vi "Update Waypoint Marker Position.vi"(8 "Error In":errorcluster, 10 "index":i32, 11 "This VI":refnum<vi>) -> (0 "error out":errorcluster)   [LabVIEW 2014]
uses:
  C:/Robotic Systems/Products/AgFalcon/Software/Ground Station/Data/Mapping DLL/GMap.NET.WindowsForms.dll
  Data/Mapping DLL/GMap.NET.WindowsForms.dll
  Reference/SubVI/Main Map Control Refernce.vi
  Missions/FGVs/Virtual Waypoints/Methods/Get Selected Virtual WP.vi
  Missions/FGVs/Virtual Waypoints/Methods/Set Selected Virtual WP.vi
  Reference/SubVI/GMap DLL Refernce.vi
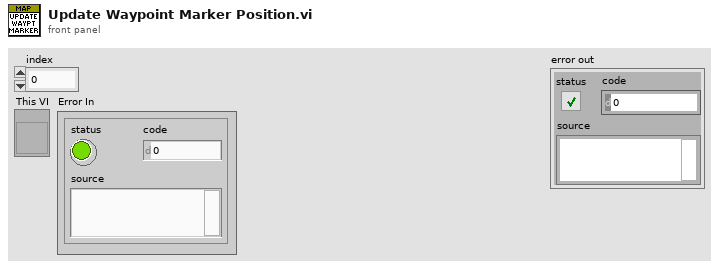
[diagram p1: front panel]
types:
  T1 = typedef "Virtual Waypoint.ctl" = cluster{"Waypoint Type":T2, "Lat":sgl, "Lon":sgl, "Altitude (m)":sgl, "Inspection Height (m)":sgl, "Circumnavigate Radius (m)":sgl, "Grid Waypoint?":bool, "Capture Photo":bool, "Speed (m/s)":sgl}
  T2 = typedef "Waypoint Type.ctl" = enum16{"PASS-THROUGH", "INSPECT", "CIRCUMNAVIGATE"}
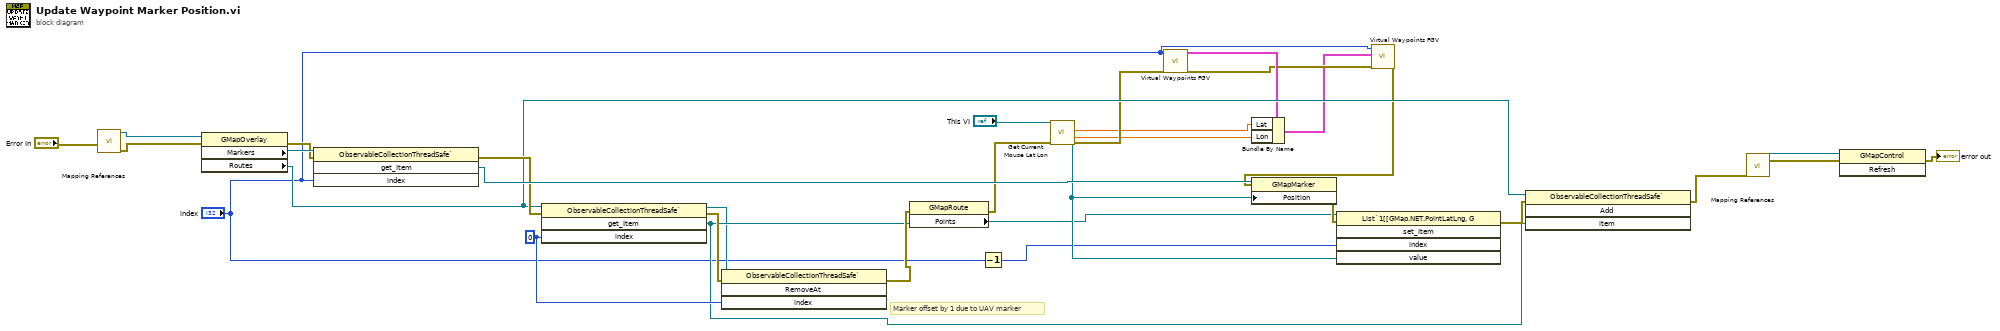
[diagram p0: block diagram]
diagram:
  w18 = 0 ("index")
  # "Marker offset by 1 due to UAV marker"
  n1 = call-poly "Mapping References.vi"("Error In"="Error In") -> ("Error Out"=w31:errorcluster, "Main Map Reference"=w32:refnum<k24>)  [unwired: 9 in]
  n2 = property class="GMapOverlay"(reference=w32, error in=w31) -> (error out=w29:errorcluster, "Markers"=w30:refnum<k24>, "Routes"=w9:refnum<k24>)  [unwired: 1 out]
  n3 = invoke class="ObservableCollectionThreadSafe`" method="get_Item"(reference=w30, error in=w29, "index"="index") -> (error out=w25:errorcluster, "get_Item"=w26:refnum<k24>)  [unwired: 1 in, 2 out]
  n4 = invoke class="ObservableCollectionThreadSafe`" method="get_Item"(reference=w9, error in=w25, "index"=w18) -> (reference out=w10:refnum<k24>, error out=w14:errorcluster, "get_Item"=w11:refnum<k24>)  [unwired: 1 in, 1 out]
  n5 = invoke class="ObservableCollectionThreadSafe`" method="RemoveAt"(reference=w10, error in=w14, "index"=w18) -> (error out=w17:errorcluster)  [unwired: 1 in, 3 out]
  n6 = property class="GMapRoute"(reference=w11, error in=w17) -> (error out=w24:errorcluster, "Points"=w21:refnum<k24>)  [unwired: 1 out]
  n7 = Decrement(x="index") -> (x-1=w20:i32)
  n8 = call "Get Current Mouse Lat Lon.vi"("error in (no error)"=w24, "This VI"="This VI") -> ("Error Out"=w8:errorcluster, "Lon"=w5:dbl, "Lat"=w6:dbl, "Point Ref"=w22:refnum<k24>)  [unwired: 6 in]
  n9 = call-poly "Virtual Waypoints FGV.vi"("Error In"=w8, "Waypoint Number"="index") -> ("Error Out"=w3:errorcluster, "Virtual Waypoint out"=w7:T1)  [unwired: 8 in]
  n10 = Bundle By Name(cluster=w7, "Lat"=w6, "Lon"=w5) -> (w2:T1)
  n11 = call-poly "Virtual Waypoints FGV.vi"("Error In"=w3, "Virtual Waypoints In"=w2, "Waypoint Index"="index") -> ("Error Out"=w1:errorcluster)  [unwired: 8 in]
  n12 = property class="GMapMarker"(reference=w26, error in=w1, "Position"=w22) -> (error out=w23:errorcluster)  [unwired: 1 out]
  n13 = invoke class="List`1[[GMap.NET.PointLatLng, G" method="set_Item"(reference=w21, error in=w23, "index"=w20, "value"=w22) -> (error out=w13:errorcluster)  [unwired: 1 in, 4 out]
  n14 = invoke class="ObservableCollectionThreadSafe`" method="Add"(reference=w9, error in=w13, "item"=w11) -> (error out=w12:errorcluster)  [unwired: 1 in, 3 out]
  n15 = call-poly "Mapping References.vi"("Error In"=w12) -> ("Error Out"=w16:errorcluster, "GMap DLL Reference"=w15:refnum<k24>)  [unwired: 9 in]
  n16 = invoke class="GMapControl" method="Refresh"(reference=w15, error in=w16) -> (error out=→"error out":errorcluster)  [unwired: 1 in, 2 out]
